vi "WPI_CompressorControlLoopCRACKED.vi"(8 "error in (no error)":errorcluster, 10 "CompressorDevRef 2":T1={"DevStatus"={"status"=FALSE, "code"=0, "source"=""}, "DigitalInputDevRef"={"DevStatus"={"status"=FALSE, "code"=0, "source"=""}, "DIO Channel"=enum."Invalid", "Digital Module"=enum."Digital Module 1"}, "RelayDevRef"={"DevStatus"={"status"=FALSE, "code"=0, "source"=""}, "Relay Channel"=enum."Invalid", "Digital Module"=enum."Digital Module 1", "Relay Direction"=enum."Both directions"}}, 11 "CompressorDevRef":T1={"DevStatus"={"status"=FALSE, "code"=0, "source"=""}, "DigitalInputDevRef"={"DevStatus"={"status"=FALSE, "code"=0, "source"=""}, "DIO Channel"=enum."Invalid", "Digital Module"=enum."Digital Module 1"}, "RelayDevRef"={"DevStatus"={"status"=FALSE, "code"=0, "source"=""}, "Relay Channel"=enum."Invalid", "Digital Module"=enum."Digital Module 1", "Relay Direction"=enum."Both directions"}}) -> ()   [LabVIEW 2012]
doc: "Monitors the pressure switch and updates the relay of up to two compressors. Use the Start, Stop, and GetEnableState VIs to update the compressor state. Use this VI in parallel with the rest of the robot code. Do not place this VI in another loop or in the Teleop code.\n\nThis software is licensed. Open the labview\\readme\\WPI Robotics Library Open Source License.txt file for more information."
uses:
  <vilib>/Rock Robotics/WPI/Compressor/WPI_CompressorDevRef.ctl
  <vilib>/Rock Robotics/WPI/DigitalInput/WPI_DigitalInputDevRef.ctl
  <vilib>/Rock Robotics/SystemInterfaces/DIO/FPGA_DIOChannel.ctl
  <vilib>/Rock Robotics/SystemInterfaces/Typedef/FPGA_TypedefDigitalModule.ctl
  <vilib>/Rock Robotics/WPI/Relay/WPI_RelayDevRef.ctl
  <vilib>/Rock Robotics/SystemInterfaces/DIO/FPGA_DIORelayChannel.ctl
  <vilib>/Rock Robotics/WPI/Relay/WPI_RelayDirection.ctl
  <vilib>/Rock Robotics/WPI/Relay/WPI_RelayValue.ctl
panel:
  # "This VI loops and doesn't return.\nPlacing it into another loop will\nprevent that loop from iterating.\n\nPeriodic tasks is a good location for it."
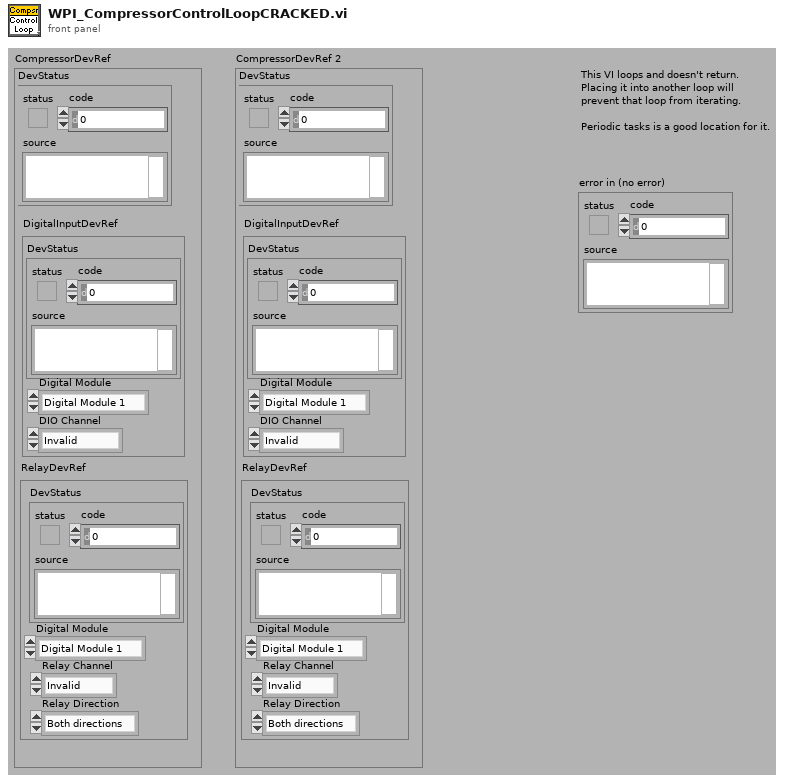
[diagram p1: front panel]
types:
  T1 = typedef "WPI_CompressorDevRef.ctl" = cluster{"DevStatus":errorcluster, "DigitalInputDevRef":T2, "RelayDevRef":T5}
  T2 = typedef "WPI_DigitalInputDevRef.ctl" = cluster{"DevStatus":errorcluster, "DIO Channel":T3, "Digital Module":T4}
  T3 = typedef "FPGA_DIOChannel.ctl" = enum8{"DIO 1", "DIO 2", "DIO 3", "DIO 4", "DIO 5", "DIO 6", "DIO 7", "DIO 8", "DIO 9", "DIO 10", "DIO 11", "DIO 12", "DIO 13", "DIO 14", "Invalid"}
  T4 = typedef "FPGA_TypedefDigitalModule.ctl" = enum16{"Digital Module 1", "Digital Module 2"}
  T5 = typedef "WPI_RelayDevRef.ctl" = cluster{"DevStatus":errorcluster, "Relay Channel":T6, "Digital Module":T4, "Relay Direction":T7}
  T6 = typedef "FPGA_DIORelayChannel.ctl" = enum8{"Relay 1", "Relay 2", "Relay 3", "Relay 4", "Relay 5", "Relay 6", "Relay 7", "Relay 8", "Invalid"}
  T7 = typedef "WPI_RelayDirection.ctl" = enum16{"Both directions", "Forward only", "Reverse only"}
  T8 = typedef "WPI_RelayValue.ctl" = enum16{"Off", "On", "Forward", "Reverse"}
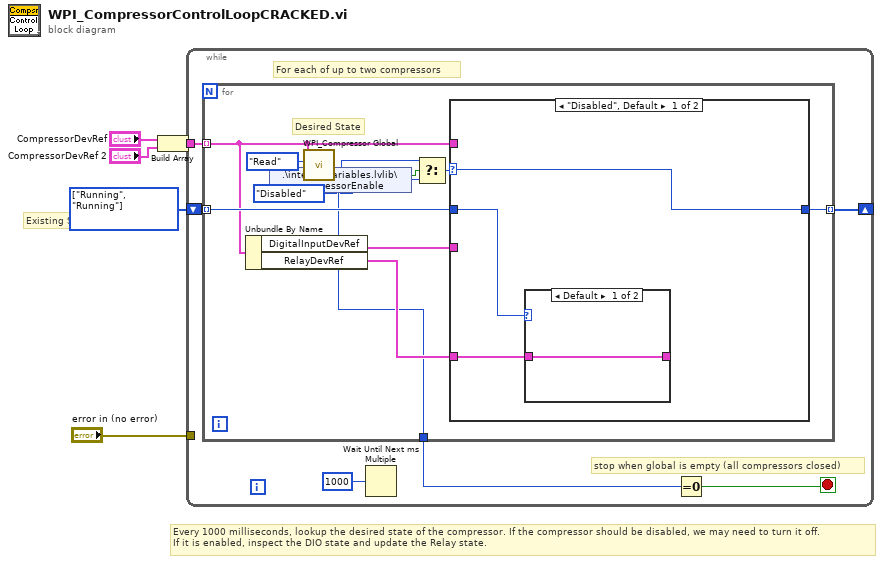
[diagram p0: block diagram]
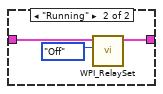
[diagram p2: hidden frame]
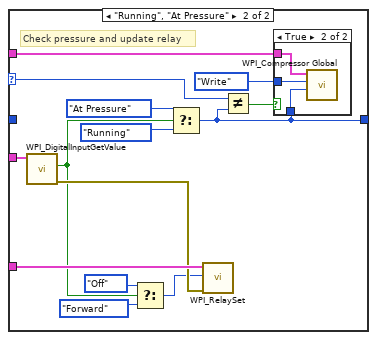
[diagram p3: hidden frame]
diagram:
  w1 = enum16{"Disabled", "Running", "At Pressure"}[] [enum."Running", enum."Running"] items=["Disabled", "Running", "At Pressure"]
  # "Every 1000 milliseconds, lookup the desired state of the compressor. If the compressor should be disabled, we may need to turn it off.\nIf it is enabled, inspect the DIO state and update the Relay state."
  # "Existing State"
  n1 = Build Array("CompressorDevRef", "CompressorDevRef 2") -> (w4:T1[])
  n2 = while {
    shift-right: [w9] -> _
    shift-left: w1 -> [w10]
    tunnel: "error in (no error)" -> [_]
    tunnel: w4 -> [w8]
    stop <- w6 stop-if-true
    # "stop when global is empty (all compressors closed)"
    # "For each of up to two compressors"
    n3 = for {
      tunnel: w10 -> [w22] mode=indexing
      tunnel: [w21] -> w9 mode=indexing
      tunnel: w8 -> [w16] mode=indexing
      tunnel: [w17] -> w7
      # "Desired State"
      n4 = Unbundle By Name(w16) -> ("DigitalInputDevRef"=w19:T2, "RelayDevRef"=w18:T5)
      n5 = shared-variable ".\\internalVariables.lvlib\\compressorEnable"() -> (w12:bool)  [unwired: 1 in, 1 out]
      n6 = call <vilib>:"WPI_Compressor Global.vi"("Operation"=enum16{"Read", "Write", "Add", "Remove"}."Read", "CompressorDevRef"=w16) -> ("Compressor State Out"=w14:enum16{"Disabled", "Running", "At Pressure"}, "Compressor Count"=w17:u8)  [unwired: 8 in]
      n7 = Select(t=w14, s=w12, f=enum16{"Disabled", "Running", "At Pressure"}."Disabled" ("t")) -> (s? t:f=w15:enum16{"Disabled", "Running", "At Pressure"})
      n8 = case shown="\"Disabled\", Default" w15 {
        selector: w15 -> [w23 w30]
        tunnel: w19 -> [_ w43]
        tunnel: w18 -> [w25 w42]
        tunnel: w22 -> [w24 _]
        tunnel: [w23 w31] -> w21
        tunnel: w16 -> [_ w33]
        frame "Disabled", Default {
          n9 = case shown="Default" w24 {
            tunnel: w25 -> [w26 w28]
            tunnel: [w26 w27] -> _
            frame Default {
            }
            frame "Running" {
              n10 = call <vilib>:"WPI_RelaySet.vi"("RelayValue"=WPI_RelayValue."Off", "RelayDevRef"=w28) -> ("RelayDevRef"=w27:T5)  [unwired: 1 in, 8 out]
            }
          }
        }
        frame "Running", "At Pressure" {
          # "Check pressure and update relay"
          n11 = call <vilib>:"WPI_DigitalInputGetValue.vi"("DigitalInputDevRef"=w43) -> ("error out"=w41:errorcluster, "Value"=w37:bool)  [unwired: 1 in, 8 out]
          n12 = Select(t=WPI_RelayValue."Off" ("RelayValue"), s=w37, f=WPI_RelayValue."Forward" ("RelayValue")) -> (s? t:f=w38:T8)
          n13 = Select(t=enum16{"Disabled", "Running", "At Pressure"}."At Pressure" ("Compressor State"), s=w37, f=enum16{"Disabled", "Running", "At Pressure"}."Running" ("Compressor State")) -> (s? t:f=w31:enum16{"Disabled", "Running", "At Pressure"})
          n14 = call <vilib>:"WPI_RelaySet.vi"("error in (no error)"=w41, "RelayValue"=w38, "RelayDevRef"=w42) -> ()  [unwired: 9 out]
          n15 = Not Equal?(x=w30, y=w31) -> (x != y?=w32:bool)
          n16 = case shown="True" w32 {
            tunnel: w31 -> [_ w46]
            tunnel: enum16{"Read", "Write", "Add", "Remove"}."Write" ("Operation") -> [_ w45]
            tunnel: w33 -> [_ w44]
            frame False {
            }
            frame True {
              n17 = call <vilib>:"WPI_Compressor Global.vi"("Compressor State In"=w46, "Operation"=w45, "CompressorDevRef"=w44) -> ()  [unwired: 7 in, 2 out]
            }
          }
        }
      }
    }
    n18 = Wait Until Next ms Multiple(millisecond multiple=u32 1000 ("timeout in ms (0)")) -> ()  [unwired: 1 out]
    n19 = Equal To 0?(x=w7) -> (x = 0?=w6:bool)
  }
